vi "Ramp 332.vi"(0 "On":bool, 1 "K/min":dbl=0.1 min=0.1 max=100.0 step=0.1 format="%.2f") -> ()   [LabVIEW 2013]
panel:
  out "Write String":string
  # "Off"
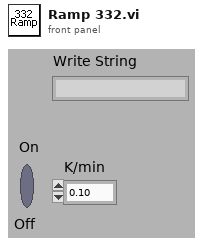
[diagram p1: front panel]
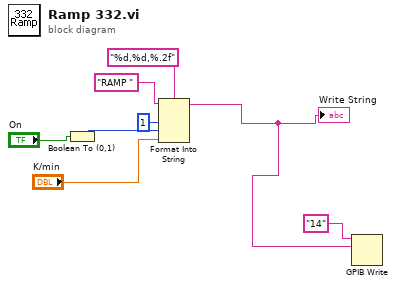
[diagram p0: block diagram]
diagram:
  n1 = Boolean To (0,1)(Boolean="On") -> (0, 1=w6:i16)
  n2 = Format Into String(format string="%d,%d,%.2f", initial string="RAMP " ("Write String"), u16 1 ("input 1"), w6, "K/min") -> (resulting string=w1:string)  [unwired: 1 in, 1 out]
  "Write String" <- w1
  n3 = GPIB Write(0:"14", 1:w1) -> ()  [unwired: 3 in, 2 out]
